vi "loggingModuleQueueFGV.vi"(8 "error in (no error)":errorcluster, 10 "message in":T2, 11 "command":T1=enum."release") -> (0 "error out":errorcluster, 2 "message out":T2)   [LabVIEW 2017, in "loggingModule.lvlib"]
uses:
  loggingModule.lvlib
  TypeDefs/message.ctl
  TypeDefs/queueFGVState.ctl
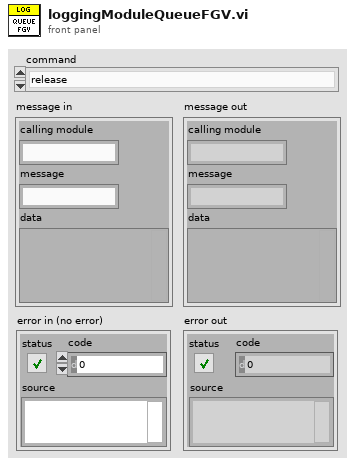
[diagram p1: front panel]
types:
  T1 = typedef "loggingModule.lvlib/queueFGVState.ctl" = enum16{"obtain", "enqueue low priority", "enqueue high priority", "dequeue", "release"}
  T2 = typedef "loggingModule.lvlib/message.ctl" = cluster{"calling module":string, "message":string, "data":variant}
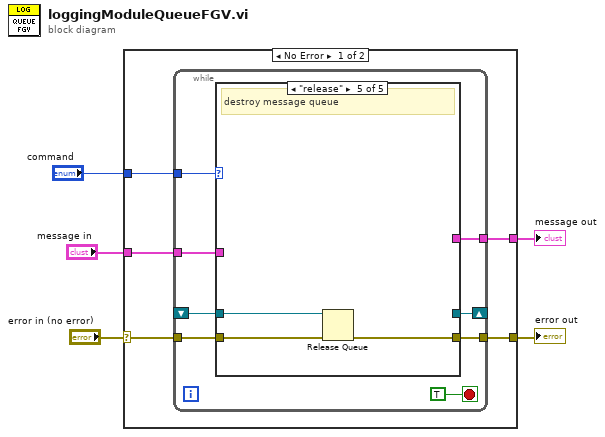
[diagram p0: block diagram]
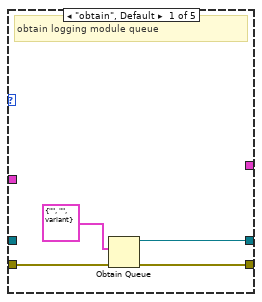
[diagram p2: hidden frame]
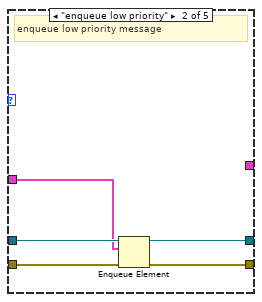
[diagram p3: hidden frame]
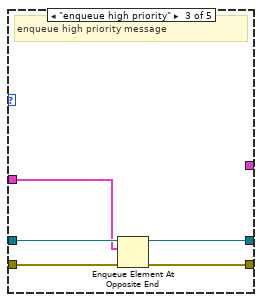
[diagram p4: hidden frame]
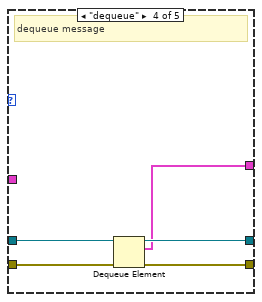
[diagram p5: hidden frame]
diagram:
  n1 = case shown="No Error" "error in (no error)" {
    selector: "error in (no error)" -> [w9 w41]
    tunnel: [w8 w41] -> w4
    tunnel: "command" -> [w10 _]
    tunnel: "message in" -> [w7 _]
    tunnel: [w6 _] -> w1
    frame No Error {
      n2 = while {
        tunnel: w10 -> [w17]
        tunnel: w9 -> [w16]
        tunnel: [w15] -> w8
        shift-right: [w14] -> _
        shift-left: _ -> [w13]
        tunnel: w7 -> [w12]
        tunnel: [w11] -> w6
        stop <- TRUE stop-if-true
        n3 = case shown="\"release\"" w17 {
          tunnel: w16 -> [w22 w27 w32 w34 w40]
          tunnel: [w21 w24 w31 w35 w38] -> w15
          tunnel: [w20 w25 w30 w36 _] -> w14
          tunnel: w13 -> [_ w26 w29 w37 w39]
          tunnel: w12 -> [_ w23 w28 _ _]
          tunnel: [_ _ _ w33 _] -> w11
          frame "obtain", Default {
            # "obtain logging module queue"
            n4 = Obtain Queue(element data type=T2 {"calling module"="", "message"="", "data"=variant} ("message in"), error in (no error)=w22) -> (queue out=w20:refnum<queue>, error out=w21:errorcluster)  [unwired: 3 in, 1 out]
          }
          frame "enqueue low priority" {
            # "enqueue low priority message"
            n5 = Enqueue Element(queue=w26, element=w23, error in (no error)=w27) -> (queue out=w25:refnum<queue>, error out=w24:errorcluster)  [unwired: 1 in, 1 out]
          }
          frame "enqueue high priority" {
            # "enqueue high priority message"
            n6 = Enqueue Element At Opposite End(queue=w29, element=w28, error in (no error)=w32) -> (queue out=w30:refnum<queue>, error out=w31:errorcluster)  [unwired: 1 in, 1 out]
          }
          frame "dequeue" {
            # "dequeue message"
            n7 = Dequeue Element(queue=w37, error in (no error)=w34) -> (queue out=w36:refnum<queue>, element=w33:T2, error out=w35:errorcluster)  [unwired: 1 in, 1 out]
          }
          frame "release" {
            # "destroy message queue"
            n8 = Release Queue(queue=w39, error in (no error)=w40) -> (error out=w38:errorcluster)  [unwired: 1 in, 2 out]
          }
        }
      }
    }
    frame Error {
    }
  }
  "error out" <- w4
  "message out" <- w1
